vi "读取baud rate.vi"(8 "error in (no error)":errorcluster caption="错误输入（无错误）", 11 "串口配置输入":refnum<class "串口配置.lvclass">) -> (0 "error out":errorcluster caption="错误输出", 2 "baud rate":u32=9600 caption="波特率(9600)", 3 "串口配置输出":refnum<class "串口配置.lvclass">)   [LabVIEW 2013, in "串口配置.lvclass"]
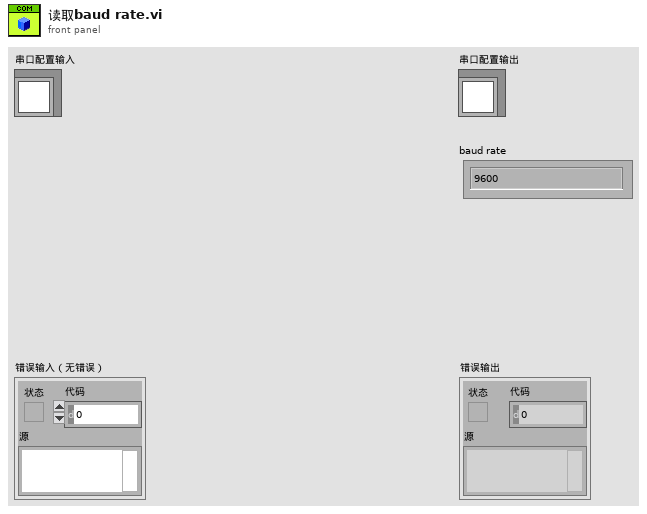
[diagram p1: front panel]
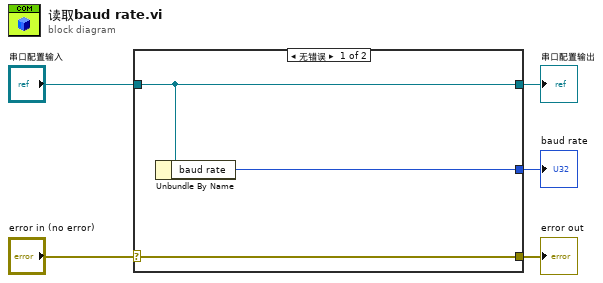
[diagram p0: block diagram]
diagram:
  n1 = case shown="无错误" "error in (no error)" {
    selector: "error in (no error)" -> [w8 w9]
    tunnel: [w8 w9] -> w4
    tunnel: [w7 w10] -> w2
    tunnel: "串口配置输入" -> [w7 w10]
    tunnel: [w6 _] -> w1
    frame No Error {
      n2 = Unbundle By Name(w7) -> ("baud rate"=w6:u32)
    }
    frame Error {
    }
  }
  "error out" <- w4
  "串口配置输出" <- w2
  "baud rate" <- w1
